vi "Create new Run Instance.vi"(7 "Kasli":string, 8 "error in":errorcluster, 9 "Script Path":path, 10 "Parameters":string[][](array[string]), 11 "Script Name":string) -> (0 "error out":errorcluster, 2 "Created?":bool, 3 "Run Instance":refnum<class "Run Instance.lvclass">)   [LabVIEW 2020, in "Run Utilities.lvlib" / "Run Instance.lvclass"]
uses:
  Run Instance.lvclass
  Support VIs/Global Memory.vi
  Interfaces/FPGA Interface/FPGA Interface.lvclass
  Run Instance.lvclass/Run Instance.ctl
  TALOS.lvlib
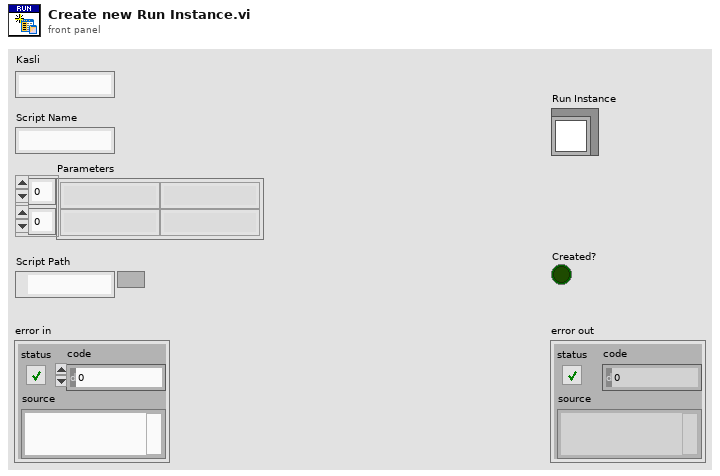
[diagram p1: front panel]
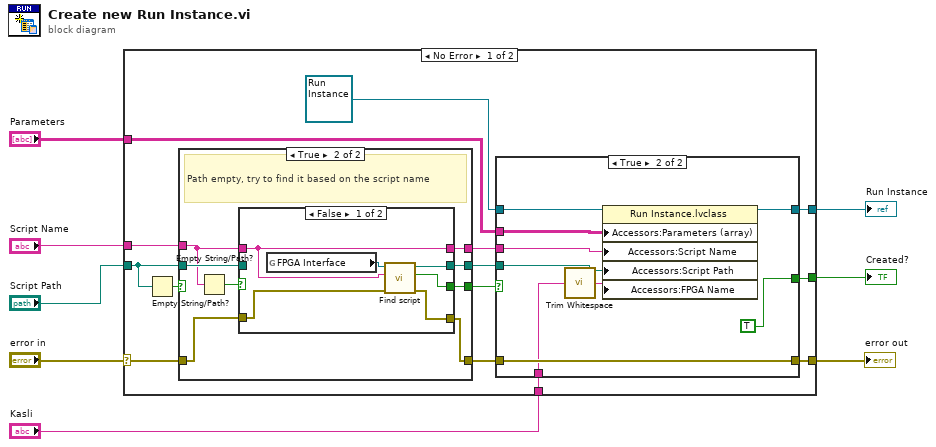
[diagram p0: block diagram]
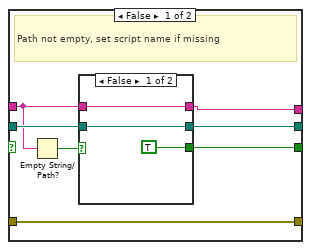
[diagram p2: hidden frame]
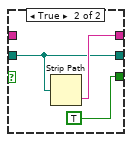
[diagram p3: hidden frame]
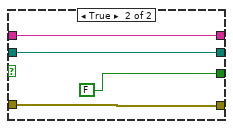
[diagram p4: hidden frame]
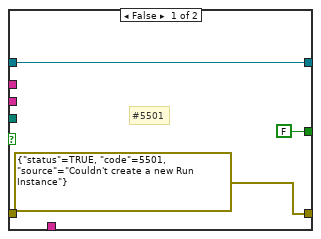
[diagram p5: hidden frame]
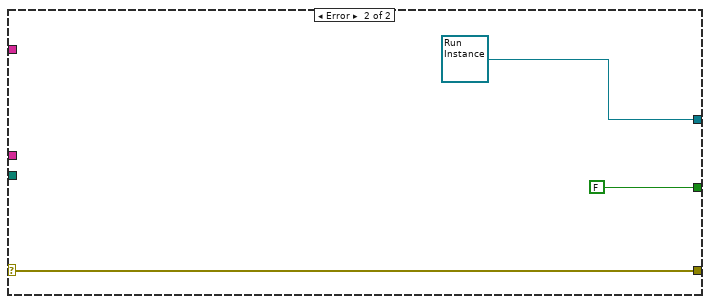
[diagram p6: hidden frame]
diagram:
  n1 = case shown="No Error" "error in" {
    selector: "error in" -> [w11 w66]
    tunnel: [w21 refnum<class "Run Instance.lvclass"> refnum ("Run Instance")] -> w7
    tunnel: "Parameters" -> [w20 _]
    tunnel: "Script Name" -> [w17 _]
    tunnel: "Script Path" -> [w15 _]
    tunnel: [w19 FALSE] -> w3
    tunnel: [w12 w66] -> w2
    tunnel: "Kasli" -> [w9 _]
    frame No Error {
      n2 = Empty String/Path?(string/path=w15) -> (empty?=w18:bool)
      n3 = case shown="True" w18 {
        tunnel: w17 -> [w24 w40]
        tunnel: [w27 w39] -> w16
        tunnel: w15 -> [w28 w42]
        tunnel: [w26 w41] -> w14
        tunnel: [w25 w38] -> w13
        tunnel: w11 -> [w23 w37]
        tunnel: [w23 w36] -> w10
        frame False {
          # "Path not empty, set script name if missing"
          n4 = Empty String/Path?(string/path=w24) -> (empty?=w29:bool)
          n5 = case shown="False" w29 {
            tunnel: w28 -> [w32 w34]
            tunnel: [w31 w35] -> w27
            tunnel: [w32 w34] -> w26
            tunnel: [TRUE TRUE] -> w25
            tunnel: w24 -> [w31 _]
            frame False {
            }
            frame True {
              n6 = Strip Path(path=w34) -> (name=w35:string)  [unwired: 1 out]
            }
          }
        }
        frame True {
          # "Path empty, try to find it based on the script name"
          n7 = Empty String/Path?(string/path=w40) -> (empty?=w43:bool)
          n8 = case shown="False" w43 {
            tunnel: w42 -> [_ w53]
            tunnel: [w49 w53] -> w41
            tunnel: w40 -> [w44 w52]
            tunnel: [w44 w52] -> w39
            tunnel: [w48 FALSE] -> w38
            tunnel: w37 -> [w46 w50]
            tunnel: [w47 w50] -> w36
            frame False {
              n9 = global read "Global Memory.vi" "FPGA Interface"() -> (w45:refnum<class "FPGA Interface.lvclass">)
              n10 = call-dynamic "Find script.vi"("error in (no error)"=w46, "Script name"=w44, "FPGA Interface"=w45) -> ("error out"=w47:errorcluster, "Found?"=w48:bool, "Script path"=w49:path)  [unwired: 6 in]
            }
            frame True {
            }
          }
        }
      }
      n11 = case shown="True" w13 {
        tunnel: refnum<class "Run Instance.lvclass"> refnum ("Run Instance") -> [w55 w64]
        tunnel: [w55 w61] -> w21
        tunnel: w20 -> [_ w63]
        tunnel: w16 -> [_ w62]
        tunnel: w14 -> [_ w59]
        tunnel: [FALSE TRUE] -> w19
        tunnel: w10 -> [_ w65]
        tunnel: [errorcluster {"status"=TRUE, "code"=5501, "source"="Couldn't create a new Run Instance"} ("error IO") w65] -> w12
        tunnel: w9 -> [_ w58]
        frame False {
          # "#5501"
        }
        frame True {
          n12 = call <vilib>:"Trim Whitespace.vi"("string"=w58) -> ("trimmed string"=w57:string)  [unwired: 1 in]
          n13 = property class="Run Instance.lvclass"(reference=w64, "Accessors:Parameters (array)"=w63, "Accessors:Script Name"=w62, "Accessors:Script Path"=w59, "Accessors:FPGA Name"=w57) -> (reference out=w61:refnum<class "Run Instance.lvclass">)  [unwired: 1 in, 1 out]
        }
      }
    }
    frame Error {
    }
  }
  "Run Instance" <- w7
  "Created?" <- w3
  "error out" <- w2
